vi "Labspec Exec.vi"(6 "Parameters":T1 items=["", "Show Style Parameters", "show single", "show overlay", "show tile", "Show Mode Parameters", "show scale fix X", "show scale fix Y", "show scale auto X", "show scale auto Y", "show scale sep x", "show scale sep y", "show scale log x", "show scale log y", "Show Axis Parameters", "axis off", "axis on"], 8 "error in":errorcluster, 9 "Command":T2 items=["Show data", "Hide data", "Remove Data", "Clone Data", "Show Style", "Show Mode", "Show Axis", "Hide all"], 10 "Data ID":i32, 11 "Automation Refnum In":refnum<k7>) -> (0 "error out":errorcluster, 1 "Clone ID":i32, 2 "Failed":bool, 3 "Automation Refnum Out":refnum<k7>)   [LabVIEW 2014]
uses:
  Exec Command.ctl
  Exec Parameters.ctl
panel:
  # "LICENSED MATERIALS – PROPERTY OF IBM\nCopyright IBM Corp. 2016,\nALL RIGHTS RESERVED"
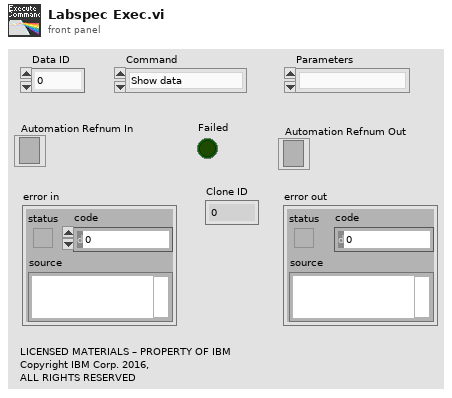
[diagram p1: front panel]
types:
  T1 = typedef "Exec Parameters.ctl" = u16
  T2 = typedef "Exec Command.ctl" = u16
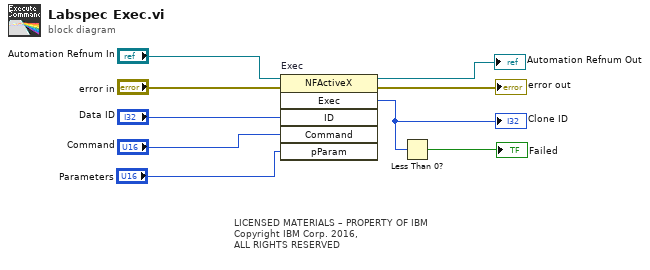
[diagram p0: block diagram]
diagram:
  # "LICENSED MATERIALS – PROPERTY OF IBM\nCopyright IBM Corp. 2016,\nALL RIGHTS RESERVED"
  n1 = invoke on="Exec" class="NFActiveX" method="Exec"(reference="Automation Refnum In", error in="error in", "ID"="Data ID", "Command"="Command", "pParam"="Parameters") -> (reference out=→"Automation Refnum Out":refnum<k7>, error out=→"error out":errorcluster, "Exec"=w2:i32)  [unwired: 1 in, 3 out]
  "Clone ID" <- w2
  n2 = Less Than 0?(x=w2) -> (x < 0?=→"Failed":bool)
